vi "5.- Prueba 5 con VISA.vi"() -> ()   [LabVIEW 2019]
uses:
  Controles/Amp_Frec.ctl
  <vilib>/Utility/error.llb/DialogType.ctl
  QMH_Support/Enqueue Message (Single).vi
  <vilib>/Utility/error.llb/Error Cluster From Error Code.vi
  <instrlib>/Pendulum CNT90/Public/Data/Read Measurement (Single).vi
  <vilib>/ErrorRing/Error Ring.xnode
  QMH_Support/Message Queue.lvlib
  QMH_Support/User Event - Stop/User Event - Stop.lvlib
  DS360/DS360.lvlib
  K2002/K2002.lvlib
  <instrlib>/Pendulum CNT90/Pendulum CNT90.lvlib
panel:
  out "mouse up?":bool
  out "EHL":i32
  out "# elements in queue":i32
  out "MHL":i32
  out "Instrumentos":i32
  in  "go_A":bool
  out "Voltaje a generar":dbl(knob) scale=0.0..10.0
  out "error out":errorcluster
  in  "stop":bool
  in  "generar":bool
  in  "Voltaje a Generar":dbl(slide)=7.0649350649350655 scale=0.0..10.0
  out "voltMon":dbl format="%.2f"
  out "frecMon":dbl format="%.2f"
  # "Ensayo Eléctrico Ponderación A"
  # "Monitoreo"
  # "Frecuencia"
  # "Hz"
  # "Voltaje"
  # "mV"
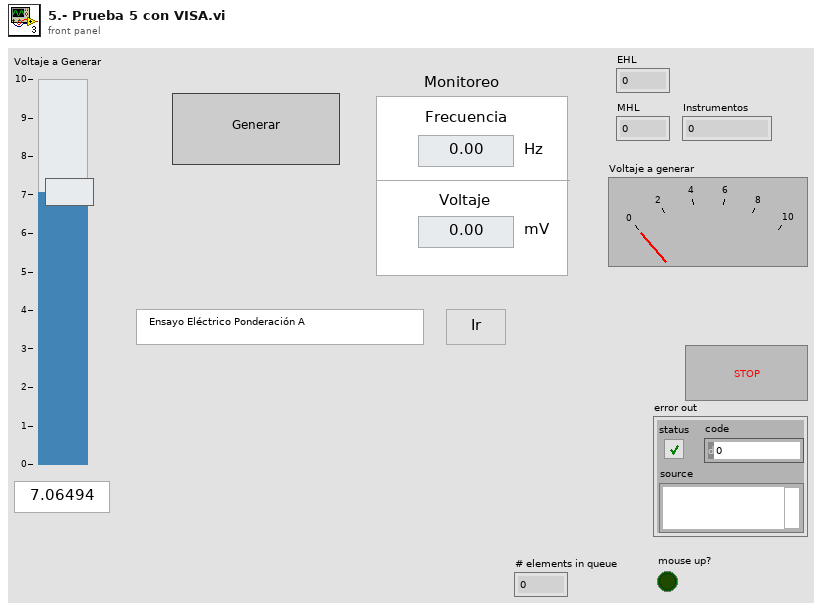
[diagram p1: front panel]
types:
  T1 = cluster{"DS360":refnum<visa-resource-name>, "K2002":refnum<visa-resource-name>, "CNT90":refnum<visa-resource-name>}
  T2 = typedef "Message Queue.lvlib/All Message Queues.ctl" = cluster{"MHL":refnum<queue>, "DS360":refnum<queue>, "K2002":refnum<queue>, "CNT90":refnum<queue>, "Instrumentos":refnum<queue>}
  T3 = typedef "Amp_Frec.ctl" = cluster{"Ampl":dbl, "Frec":dbl}
  T4 = typedef "DialogType.ctl" = u16
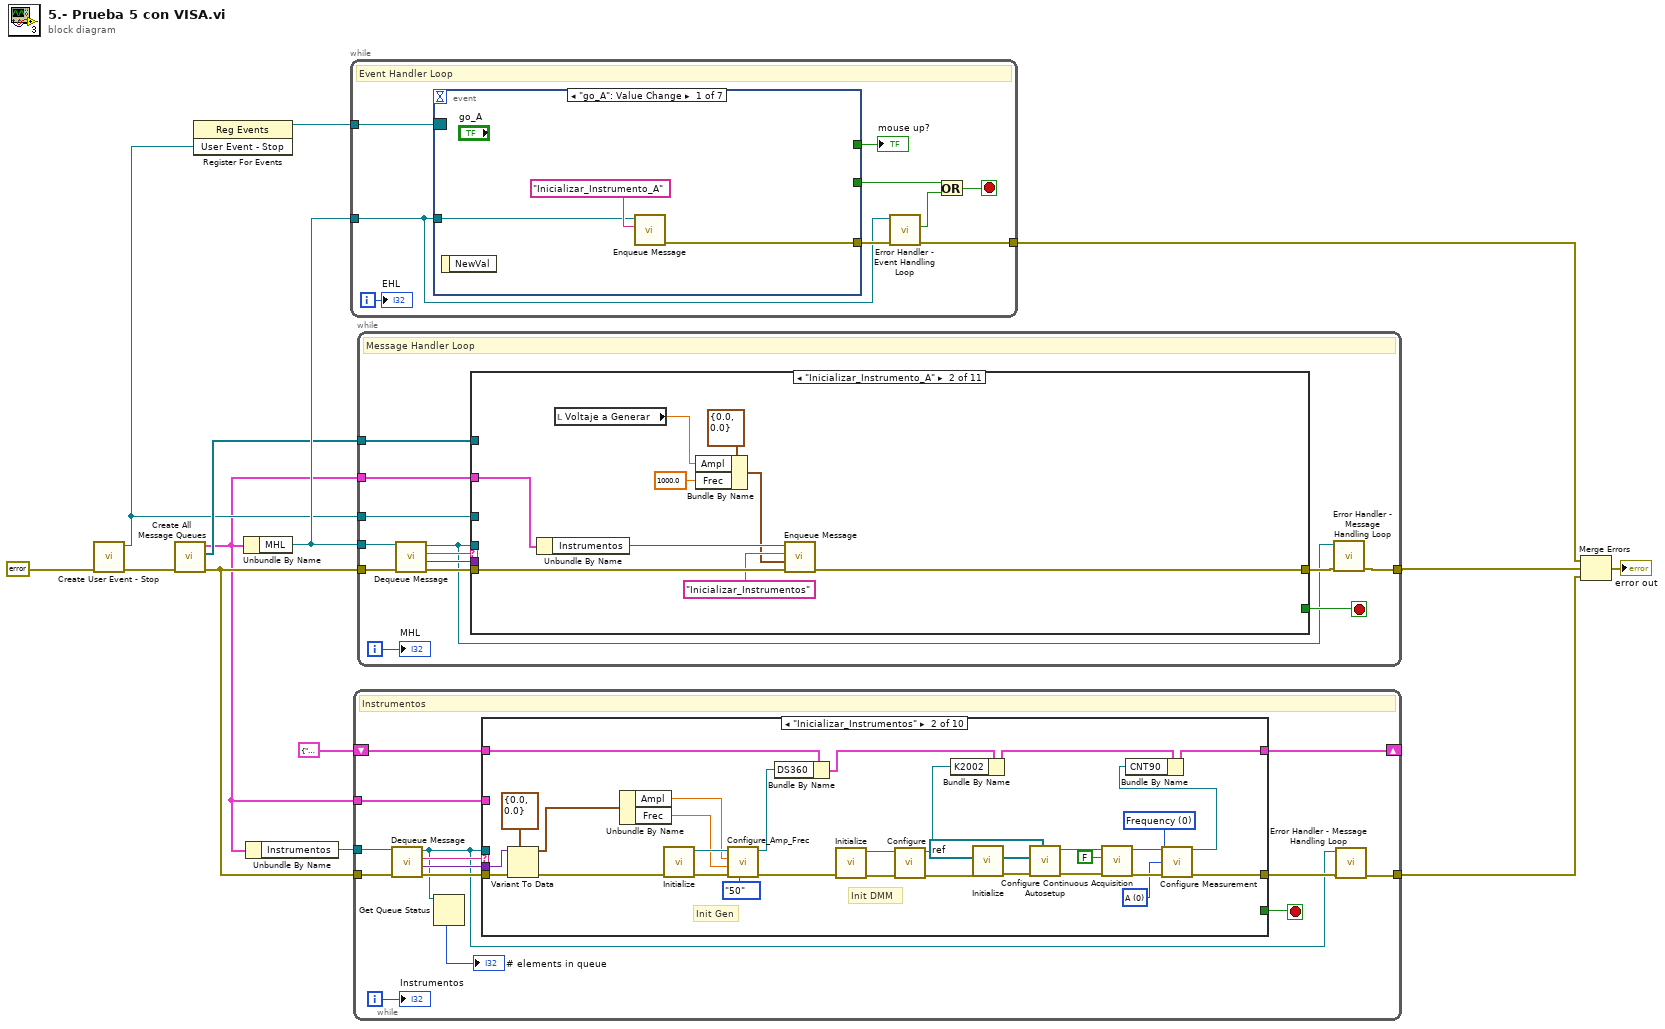
[diagram p0: block diagram]
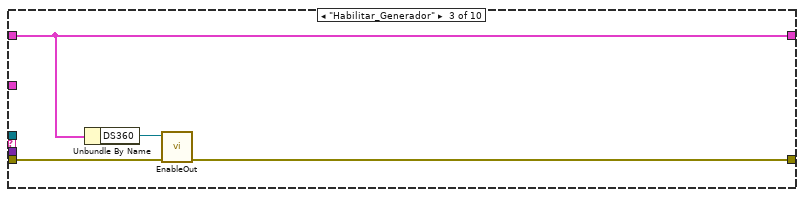
[diagram p3: hidden frame]
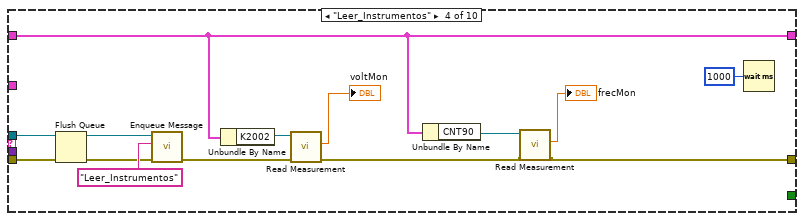
[diagram p4: hidden frame]
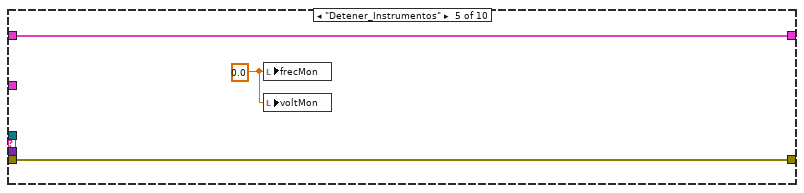
[diagram p5: hidden frame]
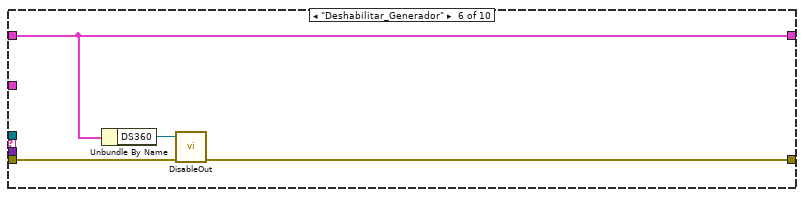
[diagram p6: hidden frame]
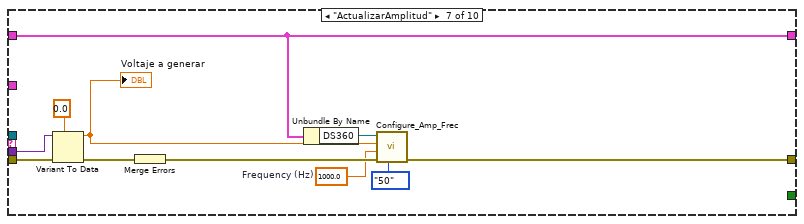
[diagram p7: hidden frame]
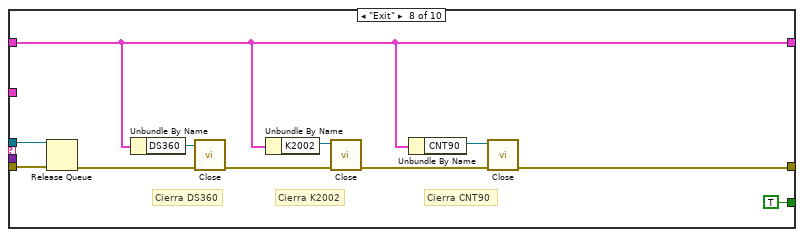
[diagram p8: hidden frame]
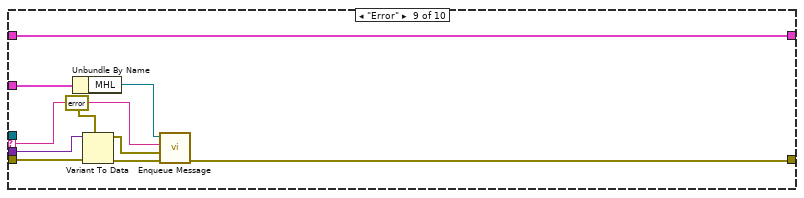
[diagram p9: hidden frame]
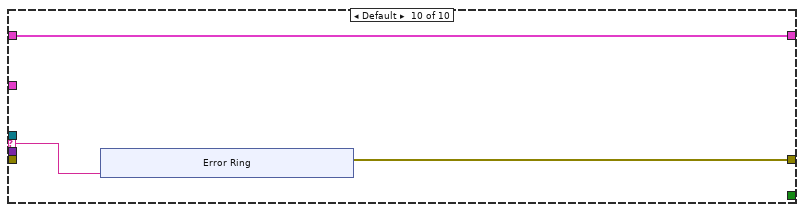
[diagram p10: hidden frame]
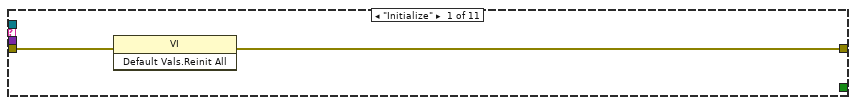
[diagram p11: hidden frame]
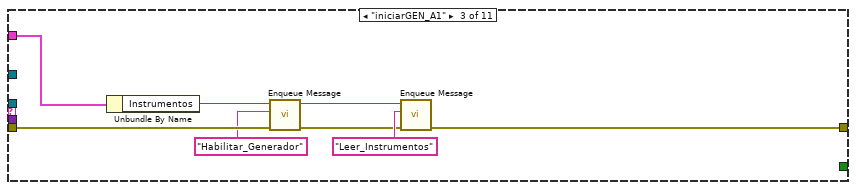
[diagram p12: hidden frame]
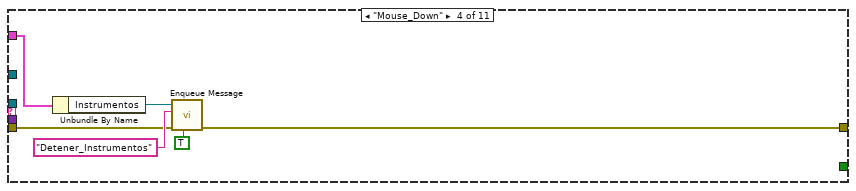
[diagram p13: hidden frame]
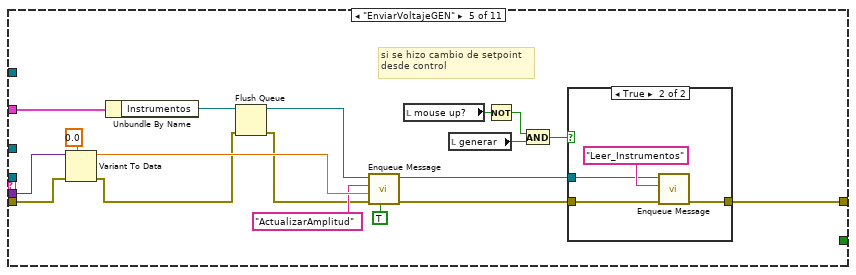
[diagram p14: hidden frame]
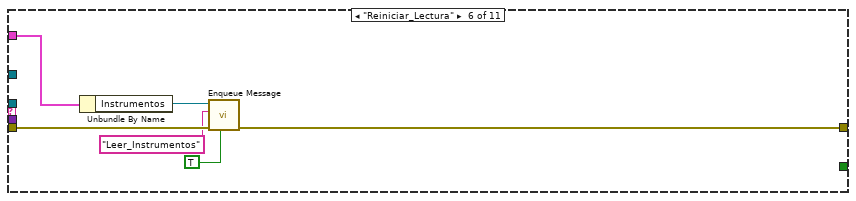
[diagram p16: hidden frame]
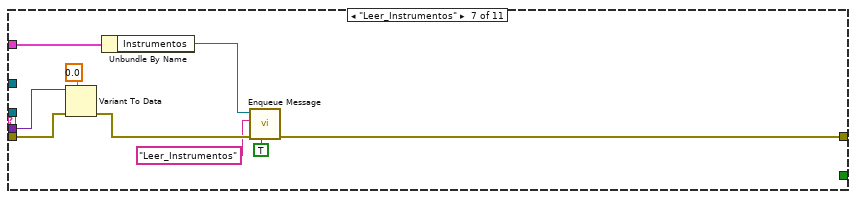
[diagram p17: hidden frame]
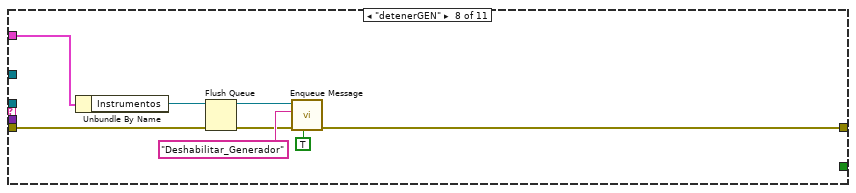
[diagram p18: hidden frame]
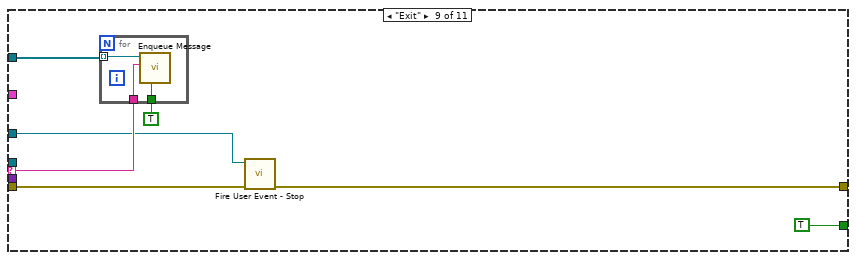
[diagram p19: hidden frame]
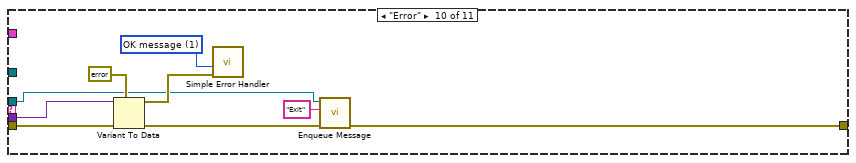
[diagram p20: hidden frame]
diagram:
  n1 = call "Create User Event - Stop.vi"("error in (no error)"=errorcluster {"status"=FALSE, "code"=0, "source"=""}) -> ("error out"=w8:errorcluster, "User Event - Stop"=w7:refnum<user-event>)  [unwired: 9 in]
  n2 = call "Create All Message Queues.vi"("error in (no error)"=w8) -> ("error out"=w4:errorcluster, "Queues Array"=w10:refnum<queue>[], "Message Queues out"=w2:T2)  [unwired: 8 in]
  n3 = register-events(w7) -> (reference out=w6:refnum<event-registration>)  [unwired: 2 in, 1 out]
  n4 = Unbundle By Name(w2) -> ("MHL"=w14:refnum<queue>)
  n5 = Unbundle By Name(w2) -> ("Instrumentos"=w5:refnum<queue>)
  n6 = while {
    tunnel: w14 -> [w20]
    tunnel: [w21] -> w13
    tunnel: w6 -> [w23]
    i -> [w16]
    stop <- w17 stop-if-true
    # "Event Handler Loop"
    n7 = event shown="[0] \"go_A\": Value Change" {
      selector: w23 -> [_ _ _ _ _ _ _]
      dyn-events: _ -> [_ _ _ _ _ _ _]
      timeout: _ -> [_ _ _ _ _ _ _]
      tunnel: w20 -> [w25 w28 w37 w43 w48 w57 _]
      tunnel: [w24 w27 w38 w42 w49 w55 _] -> w22
      tunnel: [_ _ _ _ _ _ TRUE] -> w19
      tunnel: [_ _ _ _ TRUE ("mouse up?") _ _] -> w15
      event "go_A": Value Change {
        n8 = event-data() -> ()  [unwired: 1 in, 1 out]
        n9 = call-poly "Enqueue Message.vi"("Message"="Inicializar_Instrumento_A" ("message"), "Message Queue"=w25) -> ("error out"=w24:errorcluster)  [unwired: 8 in, 1 out]
      }
      event "generar": Value Change {
        n10 = event-data() -> ("NewVal"=w29:bool)  [unwired: 1 in]
        n11 = Flush Queue(queue=w28) -> (queue out=w30:refnum<queue>, error out=w31:errorcluster)  [unwired: 1 in, 1 out]
        n12 = Select(t="iniciarGEN_A1" ("message"), s=w29, f="detenerGEN" ("message")) -> (s? t:f=w34:string)
        n13 = call-poly "Enqueue Message.vi"("Priority Message? (F)"=TRUE, "error in (no error)"=w31, "Message Data"="A1" ("message"), "Message"=w34, "Message Queue"=w30) -> ("error out"=w27:errorcluster)  [unwired: 5 in, 1 out]
      }
      event "Voltaje a Generar": Mouse Down {
        n14 = event-data() -> ()  [unwired: 1 in, 1 out]
        n15 = call-poly "Enqueue Message.vi"("Priority Message? (F)"=TRUE, "Message"="Mouse_Down" ("message"), "Message Queue"=w37) -> ("error out"=w38:errorcluster)  [unwired: 7 in, 1 out]
      }
      event "Voltaje a Generar": Value Change {
        n16 = event-data() -> ("NewVal"=w41:dbl)  [unwired: 1 in]
        n17 = call-poly "Enqueue Message.vi"("Priority Message? (F)"=TRUE, "Message Data"=w41, "Message"="EnviarVoltajeGEN" ("message"), "Message Queue"=w43) -> ("error out"=w42:errorcluster)  [unwired: 6 in, 1 out]
      }
      event "Voltaje a Generar": Mouse Up {
        n18 = event-data() -> ()  [unwired: 1 in, 1 out]
        n19 = local read "generar"() -> (w47:bool)
        n20 = case shown="True" w47 {
          tunnel: w48 -> [_ w52]
          tunnel: [errorcluster {"status"=FALSE, "code"=0, "source"=""} ("error out") w51] -> w49
          frame False {
          }
          frame True {
            n21 = call-poly "Enqueue Message.vi"("Priority Message? (F)"=TRUE, "Message"="Reiniciar_Lectura" ("message"), "Message Queue"=w52) -> ("error out"=w51:errorcluster)  [unwired: 7 in, 1 out]
          }
        }
      }
      event "stop": Value Change {
        n22 = event-data() -> ()  [unwired: 1 in, 1 out]
        n23 = call-poly "Enqueue Message.vi"("Message"="Exit", "Message Queue"=w57) -> ("error out"=w55:errorcluster)  [unwired: 8 in, 1 out]
      }
      event User Event {
        n24 = event-data() -> ()  [unwired: 1 in, 1 out]
      }
    }
    "mouse up?" <- w15
    n25 = call "Error Handler - Event Handling Loop.vi"("error in (no error)"=w22, "Message Queue"=w20) -> ("dup error in"=w21:errorcluster, "Error?"=w18:bool)  [unwired: 7 in, 1 out]
    n26 = Or(x=w19, y=w18) -> (x .or. y?=w17:bool)
    "EHL" <- w16
  }
  n27 = while {
    tunnel: w5 -> [w72]
    tunnel: w4 -> [w71]
    tunnel: [w64] -> w3
    tunnel: w2 -> [w63]
    shift-right: [w59] -> _
    shift-left: T1 {"DS360"="", "K2002"="", "CNT90"=""} -> [w60]
    i -> [w66]
    stop <- w67 stop-if-true
    # "Instrumentos"
    n28 = call "Dequeue Message.vi"("error in (no error)"=w71, "Message Queue"=w72) -> ("error out"=w70:errorcluster, "Message Data"=w68:variant, "Message"=w69:string, "dup Message Queue"=w62:refnum<queue>)  [unwired: 6 in]
    n29 = Get Queue Status(queue=w62) -> (# elements in queue=→"# elements in queue":i32)  [unwired: 2 in, 7 out]
    n30 = case shown="\"Inicializar_Instrumentos\"" w69 {
      selector: w69 -> [_ _ _ _ _ _ _ _ w158 w166]
      tunnel: w70 -> [w74 w106 w110 w122 w127 w131 w137 w153 w160 _]
      tunnel: w68 -> [_ w104 _ _ _ _ w141 _ w159 _]
      tunnel: w62 -> [_ _ _ w118 _ _ _ w152 _ _]
      tunnel: [w74 w82 w109 w113 w127 w130 w139 w145 w157 w165] -> w65
      tunnel: [_ _ _ _ _ _ _ TRUE _ _] -> w67
      tunnel: w63 -> [_ _ _ _ _ _ _ _ w156 _]
      tunnel: w60 -> [w73 w97 w107 w115 w125 w128 w133 w147 w154 w164]
      tunnel: [w73 w91 w107 w115 w125 w128 w133 w147 w154 w164] -> w59
      frame "Initialize" {
      }
      frame "Inicializar_Instrumentos" {
        w79 = 0 items=["A", "B", "C (HF-input option)", "E (Rear panel arming input)", "A prescaled by 2", "Internal Reference", "A with the variable hysteresis mode"] ("Channel  1 (0: A)")
        w80 = 0 items=["Frequency", "Burst Carrier Frequency", "Pulse Repetition Frequency", "Fall-time", "Frequency Ratio", "Positive Peak Voltage", "Negative Peak Voltage", "Negative Pulse Width", "Positive Pulse Width", "Positive Duty Cycle", "Negative Duty Cycle", "Phase", "Period", "Rise-time", "Peak-to-Peak Voltage", "Time-Interval", "Power", "Frequency Back-To-Back", "Period Back-To-Back", "TIE"] ("Measure Function (0: Frequency)")
        # "Init DMM"
        # "Init Gen"
        n31 = Variant To Data(error in=w106, type=T3 {"Ampl"=0.0, "Frec"=0.0}, Variant=w104) -> (data=w103:T3, error out=w102:errorcluster)
        n32 = Unbundle By Name(w103) -> ("Ampl"=w99:dbl, "Frec"=w98:dbl)
        n33 = call <instrlib>:"Initialize.vi"("error in (no error)"=w102) -> ("error out"=w101:errorcluster, "VISA resource name out"=w100:refnum<visa-resource-name>)  [unwired: 9 in]
        n34 = call "Configure_Amp_Frec.vi"("Impedancia"=enum16{"50", "600", "HiZ"}."50", "error in (no error)"=w101, "Frequency (Hz)"=w98, "Amplitude (Vrms)"=w99, "VISA resource name"=w100) -> ("error out"=w94:errorcluster, "VISA resource name out"=w96:refnum<visa-resource-name>)  [unwired: 5 in]
        n35 = Bundle By Name(cluster=w97, "DS360"=w96) -> (w95:T1)
        n36 = call <instrlib>:"Initialize.vi"("error in (no error)"=w94) -> ("error out"=w77:errorcluster, "VISA resource name out"=w76:refnum<visa-resource-name>)  [unwired: 9 in]
        n37 = call "Configure.vi"("error in (no error)"=w77, "VISA resource name"=w76) -> ("error out"=w89:errorcluster, "VISA resource name out"=w92:refnum<visa-resource-name>)  [unwired: 8 in]
        n38 = Bundle By Name(cluster=w95, "K2002"=w92) -> (w93:T1)
        n39 = call <instrlib>:"Initialize.vi"("error in (no error)"=w89, "VISA resource name"=refnum<visa-resource-name> "GPIB0::10::INSTR") -> ("error out"=w87:errorcluster, "VISA resource name out"=w88:refnum<visa-resource-name>)  [unwired: 8 in]
        n40 = call <instrlib>:"Autosetup.vi"("error in (no error)"=w87, "VISA resource name"=w88) -> ("error out"=w85:errorcluster, "VISA resource name out"=w86:refnum<visa-resource-name>)  [unwired: 8 in]
        n41 = call <instrlib>:"Configure Continuous Acquisition.vi"("error in (no error)"=w85, "Enable Continuous Acquisition Mode (T: True)"=FALSE, "VISA resource name"=w86) -> ("error out"=w83:errorcluster, "VISA resource name out"=w84:refnum<visa-resource-name>)  [unwired: 7 in]
        n42 = call <instrlib>:"Configure Measurement.vi"("VISA resource name"=w84, "Measure Function (0: Frequency)"=w80, "Channel  1 (0: A)"=w79, "error in (no error)"=w83) -> ("VISA resource name out"=w78:refnum<visa-resource-name>, "error out"=w82:errorcluster)  [unwired: 10 in]
        n43 = Bundle By Name(cluster=w93, "CNT90"=w78) -> (w91:T1)
      }
      frame "Habilitar_Generador" {
        n44 = Unbundle By Name(w107) -> ("DS360"=w108:refnum<visa-resource-name>)
        n45 = call "EnableOut.vi"("error in (no error)"=w110, "VISA resource name"=w108) -> ("error out"=w109:errorcluster)  [unwired: 8 in, 1 out]
      }
      frame "Leer_Instrumentos" {
        n46 = Flush Queue(queue=w118, error in (no error)=w122) -> (queue out=w117:refnum<queue>, error out=w119:errorcluster)  [unwired: 1 out]
        n47 = call-poly "Enqueue Message.vi"("error in (no error)"=w119, "Message"="Leer_Instrumentos", "Message Queue"=w117) -> ("error out"=w123:errorcluster)  [unwired: 7 in, 1 out]
        n48 = Unbundle By Name(w115) -> ("K2002"=w116:refnum<visa-resource-name>)
        n49 = call <instrlib>:"Read Measurement.vi"("error in (no error)"=w123, "VISA resource name"=w116) -> ("error out"=w114:errorcluster, "Measurement"=→"voltMon":dbl)  [unwired: 7 in, 1 out]
        n50 = Unbundle By Name(w115) -> ("CNT90"=w112:refnum<visa-resource-name>)
        n51 = call-poly <instrlib>:"Read Measurement.vi"("error in (no error)"=w114, "VISA resource name"=w112) -> ("error out"=w113:errorcluster, "Measurement"=→"frecMon":dbl)  [unwired: 7 in, 1 out]
        n52 = Wait (ms)(milliseconds to wait=u32 1000) -> ()  [unwired: 1 out]
      }
      frame "Detener_Instrumentos" {
        w126 = 0.0 ("frecMon")
        n53 = local write "frecMon"(w126) -> ()
        n54 = local write "voltMon"(w126) -> ()
      }
      frame "Deshabilitar_Generador" {
        n55 = Unbundle By Name(w128) -> ("DS360"=w129:refnum<visa-resource-name>)
        n56 = call "DisableOut.vi"("error in (no error)"=w131, "VISA resource name"=w129) -> ("error out"=w130:errorcluster)  [unwired: 8 in, 1 out]
      }
      frame "ActualizarAmplitud" {
        w135 = 1000.0  # Frequency (Hz)
        n57 = Variant To Data(error in=w137, type=0.0, Variant=w141) -> (data=w138:dbl, error out=w140:errorcluster)
        "Voltaje a generar" <- w138
        n58 = Merge Errors(w140) -> (w136:errorcluster)
        n59 = Unbundle By Name(w133) -> ("DS360"=w134:refnum<visa-resource-name>)
        n60 = call "Configure_Amp_Frec.vi"("Impedancia"=enum16{"50", "600", "HiZ"}."50", "error in (no error)"=w136, "Frequency (Hz)"=w135, "Amplitude (Vrms)"=w138, "VISA resource name"=w134) -> ("error out"=w139:errorcluster)  [unwired: 5 in, 1 out]
      }
      frame "Exit" {
        # "Cierra CNT90"
        # "Cierra K2002"
        # "Cierra DS360"
        n61 = Release Queue(queue=w152, error in (no error)=w153) -> (error out=w150:errorcluster)  [unwired: 1 in, 2 out]
        n62 = Unbundle By Name(w147) -> ("DS360"=w148:refnum<visa-resource-name>)
        n63 = call <instrlib>:"Close.vi"("error in (no error)"=w150, "VISA resource name"=w148) -> ("error out"=w149:errorcluster)  [unwired: 9 in]
        n64 = Unbundle By Name(w147) -> ("K2002"=w143:refnum<visa-resource-name>)
        n65 = call <instrlib>:"Close.vi"("error in (no error)"=w149, "VISA resource name"=w143) -> ("error out"=w146:errorcluster)  [unwired: 9 in]
        n66 = Unbundle By Name(w147) -> ("CNT90"=w144:refnum<visa-resource-name>)
        n67 = call <instrlib>:"Close.vi"("error in (no error)"=w146, "VISA resource name"=w144) -> ("error out"=w145:errorcluster)  [unwired: 9 in]
      }
      frame "Error" {
        n68 = Unbundle By Name(w156) -> ("MHL"=w155:refnum<queue>)
        n69 = Variant To Data(error in=w160, type=errorcluster {"status"=FALSE, "code"=0, "source"=""} ("error constant"), Variant=w159) -> (data=w161:errorcluster, error out=w162:errorcluster)
        n70 = call-poly "Enqueue Message.vi"("error in (no error)"=w162, "Message Data"=w161, "Message"=w158, "Message Queue"=w155) -> ("error out"=w157:errorcluster)  [unwired: 6 in, 1 out]
      }
      frame Default {
        n71 = xnode "Error Ring"("parameter 0"=w166) -> ("error out"=w165:errorcluster)
      }
    }
    n72 = call "Error Handler - Message Handling Loop.vi"("error in (no error)"=w65, "Message Queue"=w62) -> ("dup error in"=w64:errorcluster)  [unwired: 8 in, 1 out]
    "Instrumentos" <- w66
  }
  n73 = while {
    tunnel: w14 -> [w186]
    tunnel: w4 -> [w185]
    tunnel: [w177] -> w12
    tunnel: w10 -> [w181]
    tunnel: w7 -> [w179]
    tunnel: w2 -> [w175]
    i -> [w174]
    stop <- w180 stop-if-true
    # "Message Handler Loop"
    n74 = call "Dequeue Message.vi"("error in (no error)"=w185, "Message Queue"=w186) -> ("error out"=w182:errorcluster, "Message Data"=w183:variant, "Message"=w184:string, "dup Message Queue"=w176:refnum<queue>)  [unwired: 6 in]
    n75 = case shown="\"Inicializar_Instrumento_A\"" w184 {
      selector: w184 -> [_ _ _ _ _ _ _ _ w263 _ w278]
      tunnel: w183 -> [_ _ _ _ w227 _ w247 _ _ w268 _]
      tunnel: w182 -> [w188 w196 w205 w208 w228 w240 w248 w256 w260 w271 _]
      tunnel: w176 -> [_ _ _ _ _ _ _ _ _ w269 _]
      tunnel: [w187 w197 w199 w211 w217 w236 w244 w254 w259 w270 w277] -> w178
      tunnel: w181 -> [_ _ _ _ _ _ _ _ w264 _ _]
      tunnel: [_ _ _ _ _ _ _ _ TRUE _ _] -> w180
      tunnel: w179 -> [_ _ _ _ _ _ _ _ w258 _ _]
      tunnel: w175 -> [_ w194 w204 w207 w226 w239 w246 w255 _ _ _]
      frame "Initialize" {
        n76 = invoke class="VI" method="Default Vals.Reinit All"(error in=w188) -> (error out=w187:errorcluster)  [unwired: 2 in, 2 out]
      }
      frame "Inicializar_Instrumento_A" {
        n77 = Unbundle By Name(w194) -> ("Instrumentos"=w193:refnum<queue>)
        n78 = local read "Voltaje a Generar"() -> (w190:dbl)
        n79 = Bundle By Name(cluster=T3 {"Ampl"=0.0, "Frec"=0.0}, "Ampl"=w190, "Frec"=1000.0) -> (w191:T3)
        n80 = call-poly "Enqueue Message.vi"("error in (no error)"=w196, "Message Data"=w191, "Message"="Inicializar_Instrumentos", "Message Queue"=w193) -> ("error out"=w197:errorcluster)  [unwired: 6 in, 1 out]
      }
      frame "iniciarGEN_A1" {
        n81 = Unbundle By Name(w204) -> ("Instrumentos"=w203:refnum<queue>)
        n82 = call-poly "Enqueue Message.vi"("error in (no error)"=w205, "Message"="Habilitar_Generador", "Message Queue"=w203) -> ("error out"=w200:errorcluster, "dup Message Queue"=w198:refnum<queue>)  [unwired: 7 in]
        n83 = call-poly "Enqueue Message.vi"("error in (no error)"=w200, "Message"="Leer_Instrumentos", "Message Queue"=w198) -> ("error out"=w199:errorcluster)  [unwired: 7 in, 1 out]
      }
      frame "Mouse_Down" {
        n84 = Unbundle By Name(w207) -> ("Instrumentos"=w206:refnum<queue>)
        n85 = call-poly "Enqueue Message.vi"("Priority Message? (F)"=TRUE, "error in (no error)"=w208, "Message"="Detener_Instrumentos", "Message Queue"=w206) -> ("error out"=w211:errorcluster)  [unwired: 6 in, 1 out]
      }
      frame "EnviarVoltajeGEN" {
        # "si se hizo cambio de setpoint\ndesde control"
        n86 = Variant To Data(error in=w228, type=0.0, Variant=w227) -> (data=w224:dbl, error out=w220:errorcluster)
        n87 = Unbundle By Name(w226) -> ("Instrumentos"=w225:refnum<queue>)
        n88 = Flush Queue(queue=w225, error in (no error)=w220) -> (queue out=w221:refnum<queue>, error out=w219:errorcluster)  [unwired: 1 out]
        n89 = call-poly "Enqueue Message.vi"("Priority Message? (F)"=TRUE, "error in (no error)"=w219, "Message Data"=w224, "Message"="ActualizarAmplitud", "Message Queue"=w221) -> ("error out"=w218:errorcluster, "dup Message Queue"=w216:refnum<queue>)  [unwired: 5 in]
        n90 = local read "mouse up?"() -> (w213:bool)
        n91 = local read "generar"() -> (w215:bool)
        n92 = Not(x=w213) -> (.not. x?=w212:bool)
        n93 = And(x=w212, y=w215) -> (x .and. y?=w214:bool)
        n94 = case shown="True" w214 {
          tunnel: w218 -> [w230 w233]
          tunnel: [w230 w232] -> w217
          tunnel: w216 -> [_ w231]
          frame False {
          }
          frame True {
            n95 = call-poly "Enqueue Message.vi"("error in (no error)"=w233, "Message"="Leer_Instrumentos" ("message"), "Message Queue"=w231) -> ("error out"=w232:errorcluster)  [unwired: 7 in, 1 out]
          }
        }
      }
      frame "Reiniciar_Lectura" {
        n96 = Unbundle By Name(w239) -> ("Instrumentos"=w238:refnum<queue>)
        n97 = call-poly "Enqueue Message.vi"("Priority Message? (F)"=TRUE, "error in (no error)"=w240, "Message"="Leer_Instrumentos", "Message Queue"=w238) -> ("error out"=w236:errorcluster)  [unwired: 6 in, 1 out]
      }
      frame "Leer_Instrumentos" {
        n98 = Variant To Data(error in=w248, type=0.0, Variant=w247) -> (error out=w245:errorcluster)  [unwired: 1 out]
        n99 = Unbundle By Name(w246) -> ("Instrumentos"=w241:refnum<queue>)
        n100 = call-poly "Enqueue Message.vi"("Priority Message? (F)"=TRUE, "error in (no error)"=w245, "Message"="Leer_Instrumentos", "Message Queue"=w241) -> ("error out"=w244:errorcluster)  [unwired: 6 in, 1 out]
      }
      frame "detenerGEN" {
        n101 = Unbundle By Name(w255) -> ("Instrumentos"=w251:refnum<queue>)
        n102 = Flush Queue(queue=w251, error in (no error)=w256) -> (queue out=w250:refnum<queue>, error out=w252:errorcluster)  [unwired: 1 out]
        n103 = call-poly "Enqueue Message.vi"("Priority Message? (F)"=TRUE, "error in (no error)"=w252, "Message"="Deshabilitar_Generador", "Message Queue"=w250) -> ("error out"=w254:errorcluster)  [unwired: 6 in, 1 out]
      }
      frame "Exit" {
        n104 = for {
          tunnel: w264 -> [w267] mode=indexing
          tunnel: w263 -> [w266]
          tunnel: TRUE -> [w265]
          n105 = call-poly "Enqueue Message.vi"("Priority Message? (F)"=w265, "Message"=w266, "Message Queue"=w267) -> ()  [unwired: 7 in, 2 out]
        }
        n106 = call "Fire User Event - Stop.vi"("error in (no error)"=w260, "User Event - Stop"=w258) -> ("error out"=w259:errorcluster)  [unwired: 9 in]
      }
      frame "Error" {
        w275 = T4 1 items=["no dialog", "OK message", "continue or stop message", "OK message + warnings", "continue/stop + warnings"] ("type of dialog (OK msg:1)")
        n107 = Variant To Data(error in=w271, type=errorcluster {"status"=FALSE, "code"=0, "source"=""} ("error out"), Variant=w268) -> (data=w273:errorcluster, error out=w272:errorcluster)
        n108 = call <vilib>:"Simple Error Handler.vi"("type of dialog (OK msg:1)"=w275, "error in (no error)"=w273) -> ()  [unwired: 3 in, 5 out]
        n109 = call-poly "Enqueue Message.vi"("error in (no error)"=w272, "Message"="Exit", "Message Queue"=w269) -> ("error out"=w270:errorcluster)  [unwired: 7 in, 1 out]
      }
      frame Default {
        n110 = xnode "Error Ring"("parameter 0"=w278) -> ("error out"=w277:errorcluster)
      }
    }
    n111 = call "Error Handler - Message Handling Loop.vi"("error in (no error)"=w178, "Message Queue"=w176) -> ("dup error in"=w177:errorcluster)  [unwired: 8 in, 1 out]
    "MHL" <- w174
  }
  n112 = Merge Errors(w13, w12, w3) -> (→"error out":errorcluster)
